vi "LJM_eReadAddresses.vi"(0 "Handle In":i32, 1 "NumFrames":i32, 5 "aAddresses":i32[](array[numeric]), 7 "aTypes":i32[](array[numeric]), 11 "error in":errorcluster) -> (4 "Handle Out":i32, 10 "aValues":dbl[](array[numeric]) format="%.2f", 14 "ErrorAddress":i32, 15 "error out":errorcluster)   [LabVIEW 2017]
uses:
  labjackm.dll
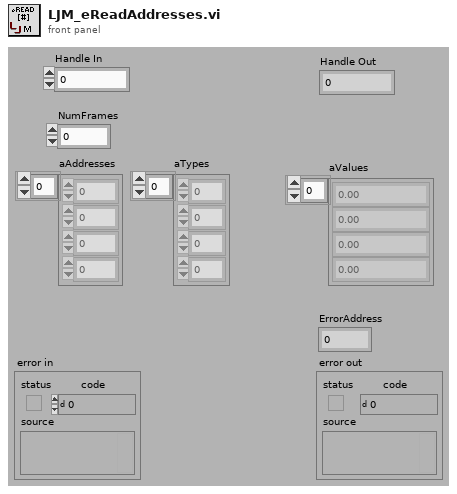
[diagram p1: front panel]
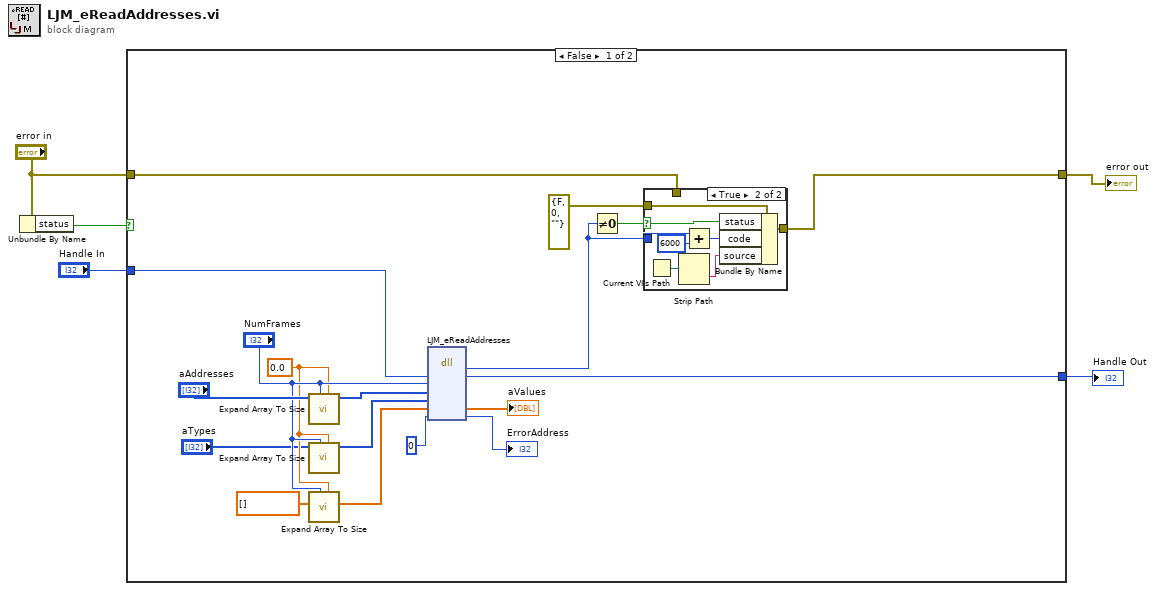
[diagram p0: block diagram]
diagram:
  n1 = Unbundle By Name("error in") -> ("status"=w5:bool)
  n2 = case shown="False" w5 {
    tunnel: "error in" -> [w20 w34]
    tunnel: [w19 w34] -> w3
    tunnel: [w7 w33] -> w2
    tunnel: "Handle In" -> [w6 w33]
    frame False {
      w15 = 0.0 ("Default Value")
      n3 = call <userlib>:"Expand Array To Size.vi"("Default Value"=w15, "# Elements"="NumFrames", "I32 Array In"="aAddresses") -> ("I32 Array Out"=w17:i32[])  [unwired: 4 in, 4 out]
      n4 = call <userlib>:"Expand Array To Size.vi"("Default Value"=w15, "# Elements"="NumFrames", "I32 Array In"="aTypes") -> ("I32 Array Out"=w13:i32[])  [unwired: 4 in, 4 out]
      n5 = call <userlib>:"Expand Array To Size.vi"("Default Value"=w15, "# Elements"="NumFrames", "DBL Array In"=dbl[] []) -> ("DBL Array Out"=w11:dbl[])  [unwired: 4 in, 4 out]
      n6 = dll-call lib="labjackm.dll" fn="LJM_eReadAddresses"("Handle"=w6, "NumFrames"="NumFrames", "aAddresses"=w17, "aTypes"=w13, "aValues"=w11, "ErrorFrame"=u32 0) -> (w23:i32, "Handle"=w7:i32, "aValues"=→"aValues":dbl[], "ErrorFrame"=→"ErrorAddress":i32)  [unwired: 6 in, 2 out]
      n7 = Not Equal To 0?(x=w23) -> (x != 0?=w22:bool)
      n8 = case shown="True" w22 {
        selector: w22 -> [_ w31]
        tunnel: [w24 w32] -> w19
        tunnel: errorcluster {"status"=FALSE, "code"=0, "source"=""} ("error IO") -> [_ w30]
        tunnel: w23 -> [_ w26]
        tunnel: w20 -> [w24 _]
        frame False {
        }
        frame True {
          n9 = Current VI's Path() -> (path=w28:path)
          n10 = Strip Path(path=w28) -> (name=w29:string)  [unwired: 1 out]
          n11 = Add(x=w26, y=6000) -> (x+y=w27:i32)
          n12 = Bundle By Name(cluster=w30, "status"=w31, "code"=w27, "source"=w29) -> (w32:errorcluster)
        }
      }
    }
    frame True {
    }
  }
  "error out" <- w3
  "Handle Out" <- w2
